vi "init odor config color ring (sub-vi).vi"(8 "error in (no error)":errorcluster, 11 "ring refnum":refnum<vi>) -> (0 "error out":errorcluster, 3 "reference out":refnum<vi>)   [LabVIEW 2021]
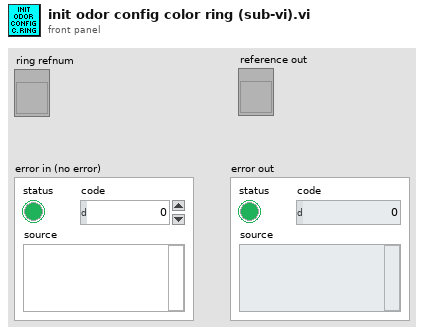
[diagram p1: front panel]
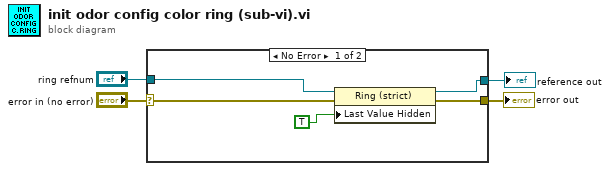
[diagram p0: block diagram]
diagram:
  n1 = case shown="No Error" "error in (no error)" {
    selector: "error in (no error)" -> [w8 w10]
    tunnel: [w9 w10] -> w4
    tunnel: "ring refnum" -> [w7 w11]
    tunnel: [w6 w11] -> w1
    frame No Error {
      n2 = property class="Ring (strict)"(reference=w7, error in=w8, "Last Value Hidden"=TRUE) -> (reference out=w6:refnum<vi>, error out=w9:errorcluster)
    }
    frame Error {
    }
  }
  "error out" <- w4
  "reference out" <- w1
